vi "HMI Panel.vi"() -> ()   [LabVIEW 2014]
uses:
  <vilib>/Platform/TimedLoop/XDataNode/timing_clust.ctl
  <vilib>/Platform/TimedLoop/XDataNode/nitl_modes.ctl
  <vilib>/Platform/TimedLoop/XDataNode/wakeup.ctl
  <vilib>/Utility/inputDevices.llb/closeJoystick.vi
  <vilib>/Utility/inputDevices.llb/joystickAcquire.vi
  <vilib>/Platform/TimedLoop/XDataNode/XDataNode.xnode
  <vilib>/Platform/TimedLoop/XDataNode/XDNodeRunTimeDep.lvlib
panel:
  out "error out 2":errorcluster
  out "data out 2":string
  out "data out":string
  out "Period":i64
  out "Finished Late? [i-1]":bool
  out "String":string
  out "error out 3":errorcluster
  out "error out":errorcluster
  in  "error in":errorcluster
  in  "error in":errorcluster
  in  "Activate Joystick":bool=TRUE
  in  "Activate Oculus Rift":bool
  in  "?":enum32{"Logiteck Joystick", "Oculus Rift"}(tab)
  in  "?":dbl
  in  "?":dbl
  in  "?":dbl
  out "Vertical":dbl(slide) scale=-100.0..100.0
  out "?":cluster{dbl[], dbl[]}[](graph)
  out "Yaw":dbl(slide) scale=-100.0..100.0
  out "?":dbl(knob) scale=0.0..360.0
  out "Joystick Status":bool
  in  "Joystick Selector":u16(ring)=1 items=["Logitech Freedom 2.4 USB"]
  out "z":dbl(slide) scale=-1.5..1.5
  out "y":dbl(slide) scale=-1.5..1.5
  out "x":dbl(slide) scale=-1.5..1.5
  in  "Operation Mode":u16(ring)=1 items=["Disabled", "Standard"]
  in  "Port Joyst.TCP":u16=6340
  out "Oculus Rift Status":bool
  in  "SYA":dbl(slide)=1.0 scale=0.0..1.0
  in  "SZR":dbl(slide)=1.0 scale=0.0..1.0
  in  "SZA":dbl(slide)=1.0 scale=0.0..1.0
  in  "SXA":dbl(slide)=1.0 scale=0.0..1.0
  out "Error Out":errorcluster
  in  "DZZR":i32(slide)=20 scale=0.0..100.0
  in  "DZZA":i32(slide)=20 scale=0.0..100.0
  in  "DZYA":i32(slide)=10 scale=0.0..100.0
  in  "DZXA":i32(slide)=10 scale=0.0..100.0
  in  "InvZA":bool=TRUE
  in  "InvYA":bool
  in  "InvXA":bool
  in  "stop":bool
  in  "Joystick Button Ref":refnum<vi>
  in  "TCPConRef":refnum<k5>
  out "direction info":T1
  out "button info":T2
  out "axis info":T3
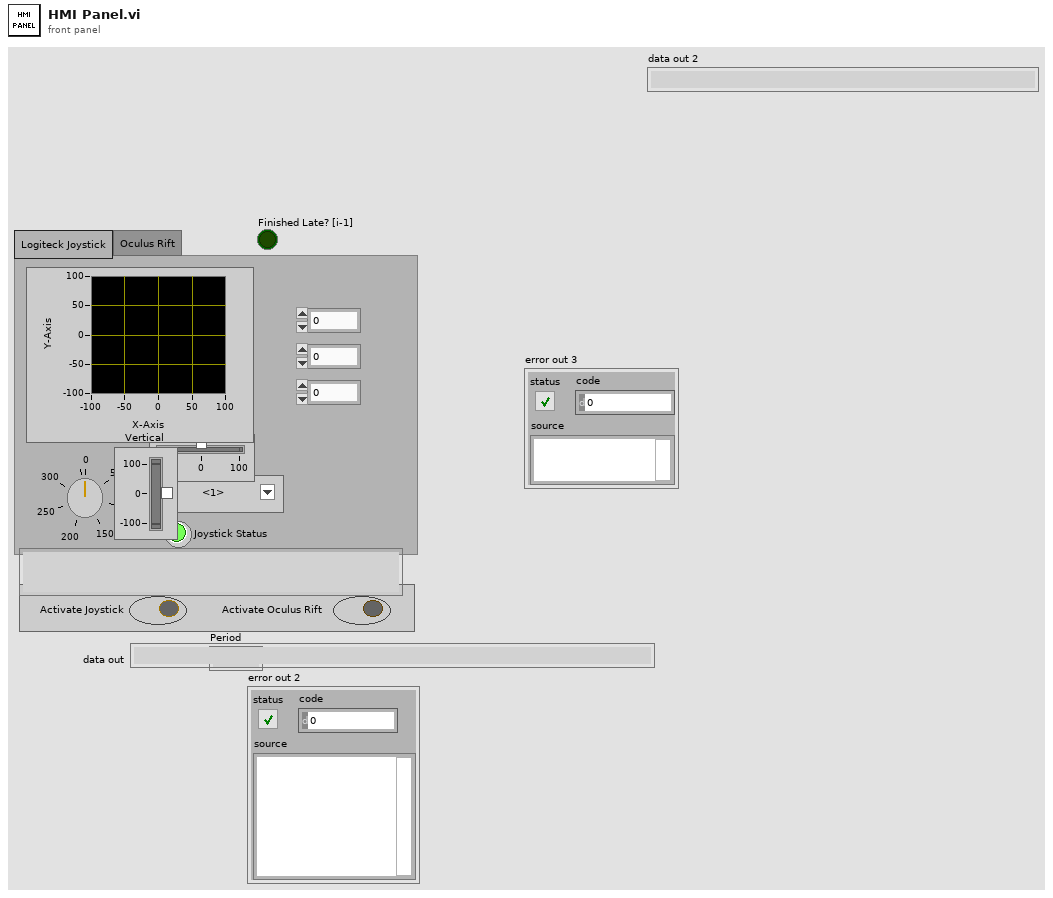
[diagram p1: front panel]
types:
  T1 = cluster{"pov 1":i32, "pov 2":i32, "pov 3":i32, "pov 4":i32}
  T2 = cluster{"button 1":bool, "button 2":bool, "button 3":bool, "button 4":bool, "button 5":bool, "button 6":bool, "button 7":bool, "button 8":bool, "button 9":bool, "button 10":bool, "button 11":bool, "button 12":bool, "button 13":bool, "button 14":bool, "button 15":bool, "button 16":bool, "button 17":bool, "button 18":bool, "button 19":bool, "button 20":bool, "button 21":bool, "button 22":bool, "button 23":bool, "button 24":bool, "button 25":bool, "button 26":bool, "button 27":bool, "button 28":bool, "button 29":bool, "button 30":bool, "button 31":bool, "button 32":bool}
  T3 = cluster{"X axis":i32, "Y axis":i32, "Z axis":i32, "X axis rotation":i32, "Y axis rotation":i32, "Z axis rotation":i32, "U axis":i32, "V axis":i32}
  T4 = typedef "XDNodeRunTimeDep.lvlib/timing_clust.ctl" = cluster{"Expected End [f-1]":u64, "Actual End [f-1]":u64, "Finished Late? [f-1]":bool, "Expected End [i-1]":u64, "Actual End [i-1]":u64, "Finished Late? [i-1]":bool, "Expected Start [i]":u64, "Actual Start [i]":u64, "Expected Start [f]":u64, "Actual Start [f]":u64, "Source Name":string, "Structure Name":string, "Period":i64, "Deadline":i64, "Offset":i64, "Start":i64, "Priority":i32, "Timeout":i32, "Mode":T5, "Wakeup Reason":T6, "Error":errorcluster, "Source Type":string, "Secondary Source Type":string, "Global End Time":u64, "Global Start Time":u64, "Frame Duration":u64, "Iteration Duration":u64, "Assigned CPU":i32, "I/O Scan Engine Mode":u32}
  T5 = typedef "XDNodeRunTimeDep.lvlib/nitl_modes.ctl" = enum32{"No Change", "Process missed periods, maintain original phase", "Discard missed periods, maintain original phase", "Process missed periods, ignore original phase", "Discard missed periods, ignore original phase"}
  T6 = typedef "XDNodeRunTimeDep.lvlib/wakeup.ctl" = enum32{"Normal", "Aborted", "Asynchronous wakeup", "Timing source error", "Timed loop error", "Timeout"}
  T7 = cluster{"axes total":u32, "buttons total":u32, "pov total":u32, "device name":string}[]
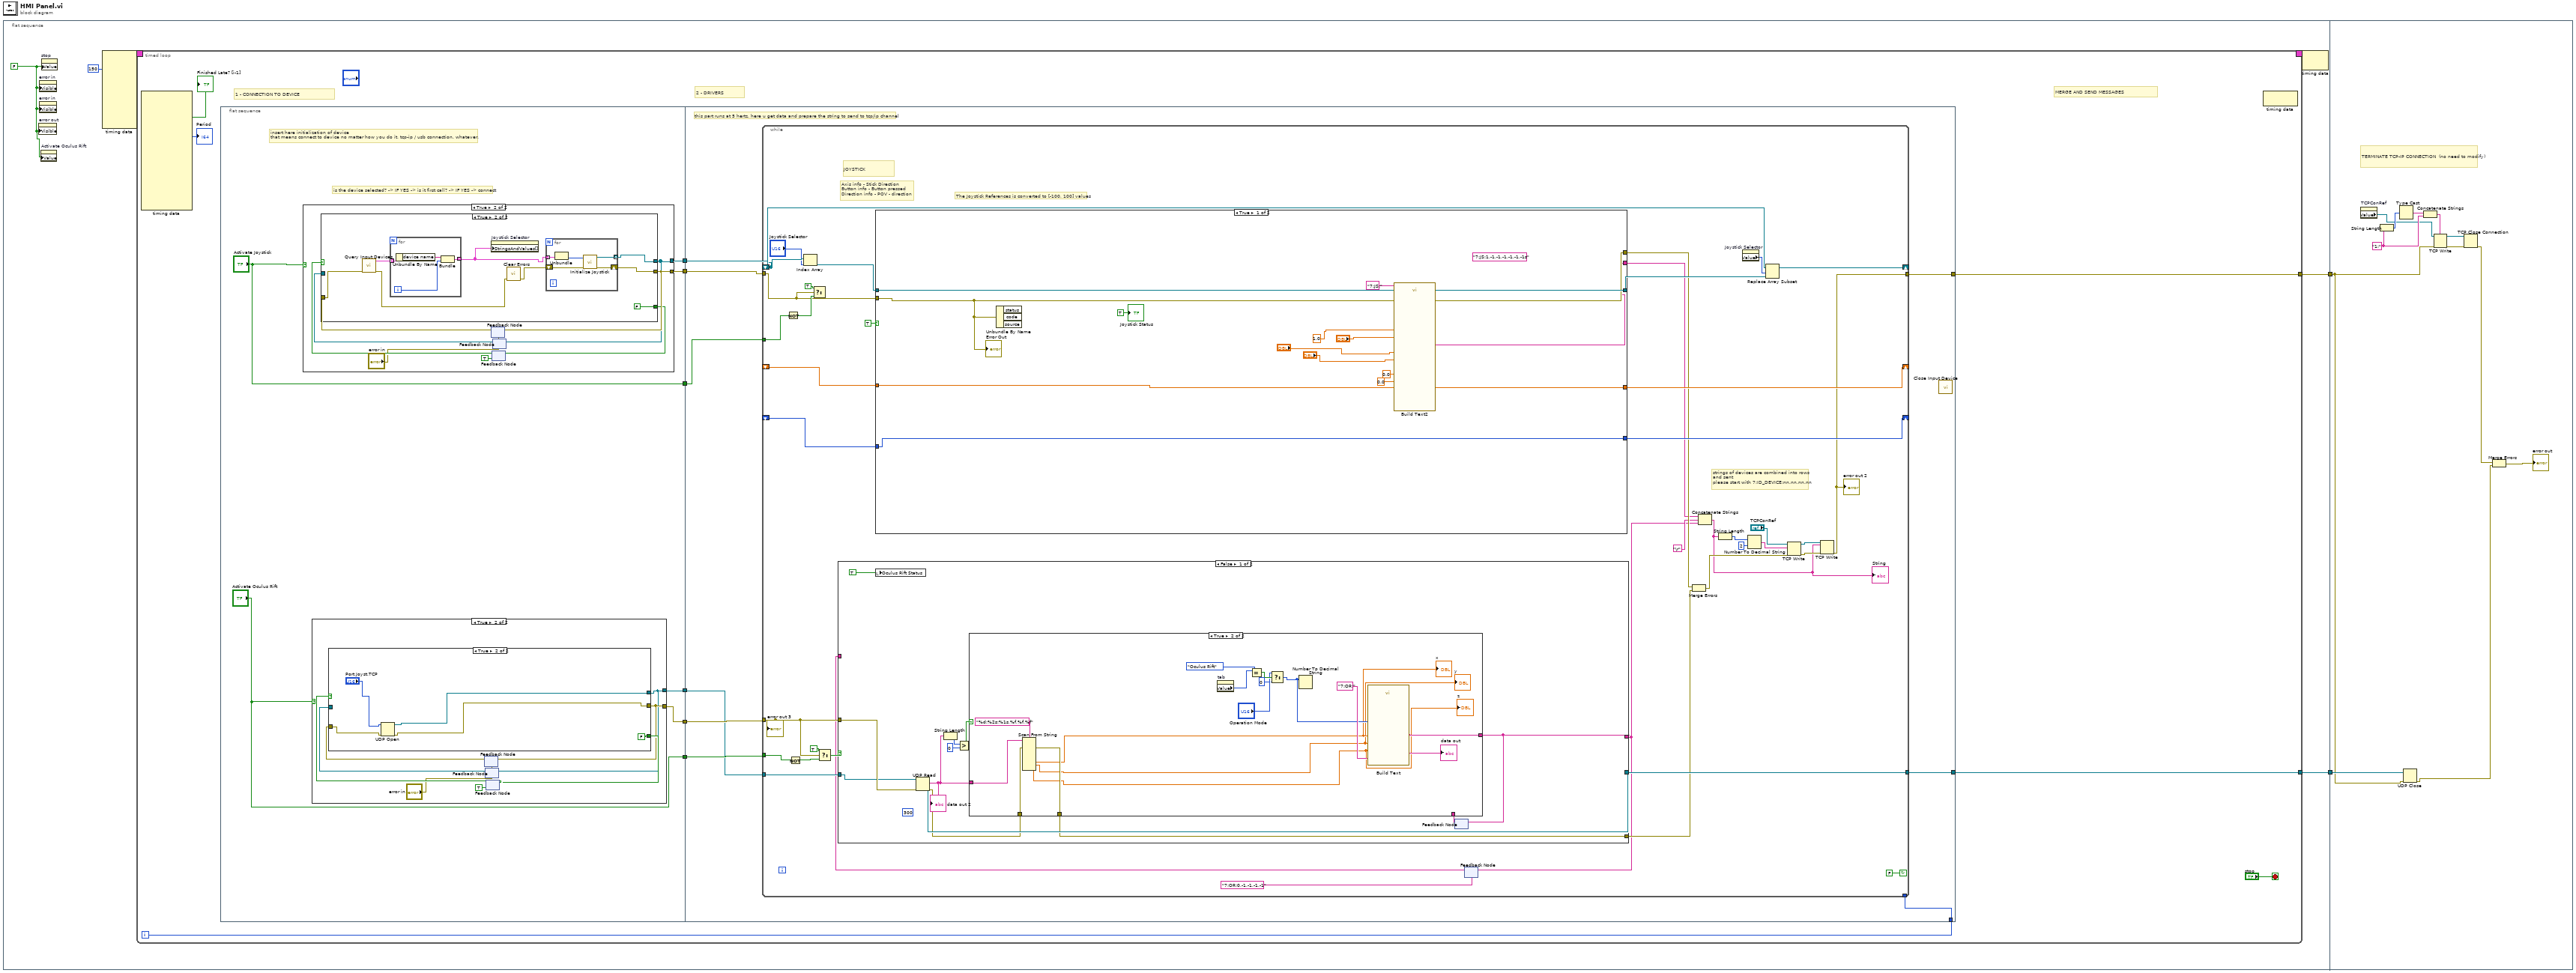
[diagram p0: block diagram]
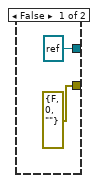
[diagram p2: hidden frame]
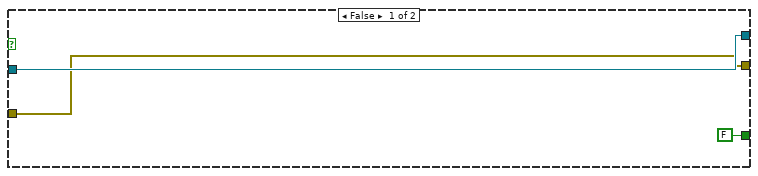
[diagram p3: hidden frame]
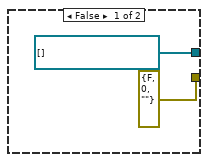
[diagram p4: hidden frame]
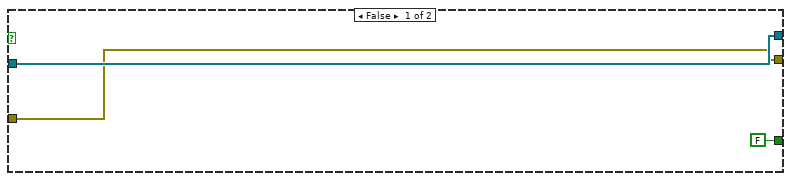
[diagram p5: hidden frame]
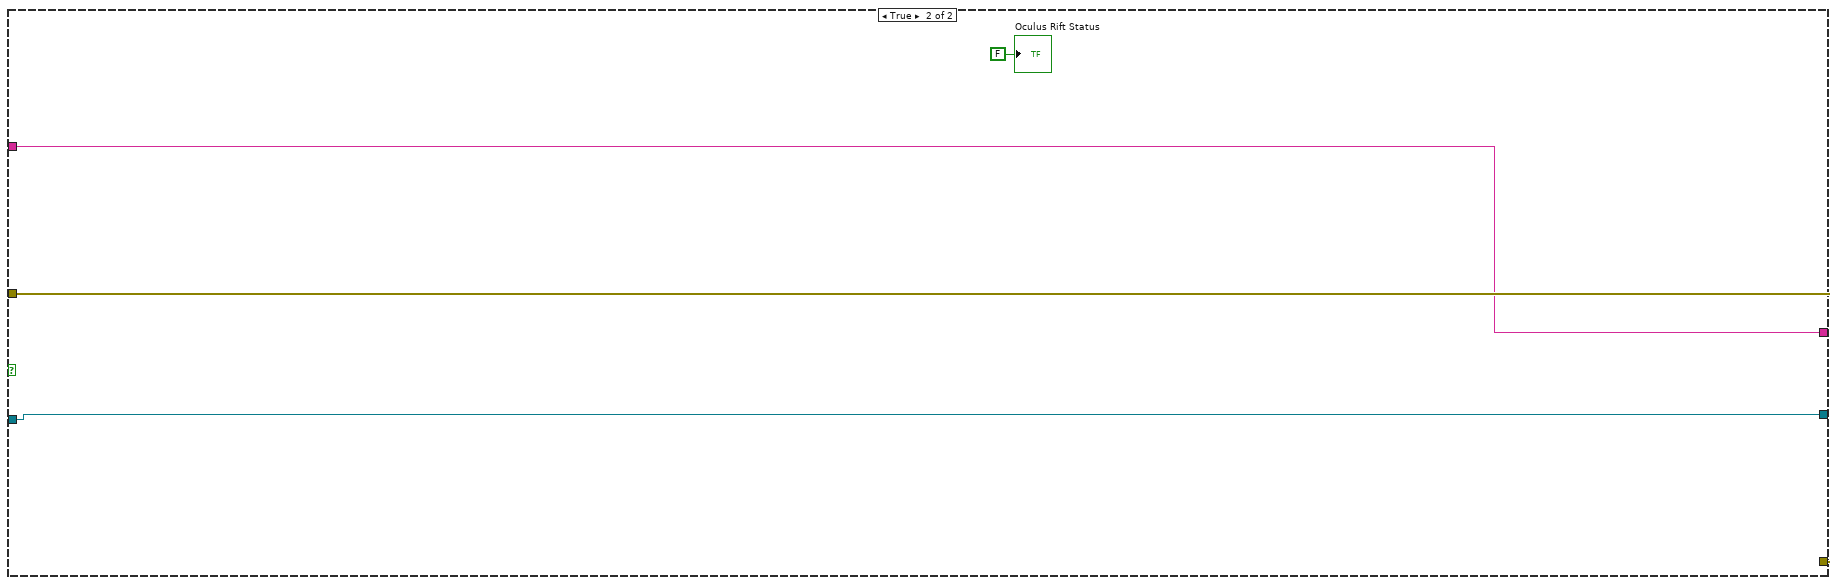
[diagram p7: hidden frame]
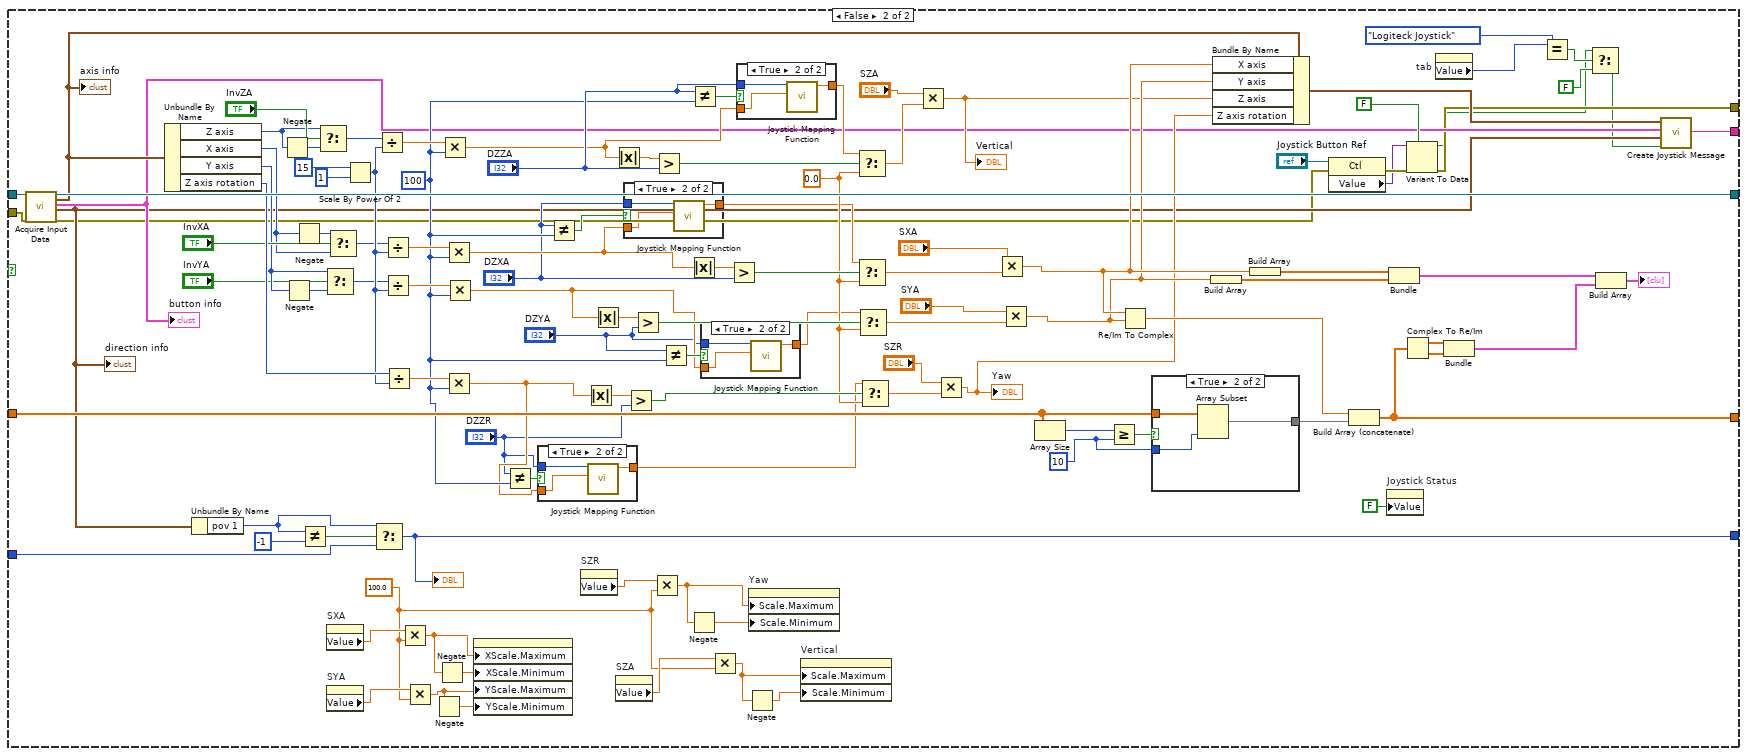
[diagram p8: hidden frame]
diagram:
  n1 = flat-sequence {
    tunnel: [w5] -> w2
    tunnel: [w4] -> w1
    tunnel: w2 -> [w310]
    tunnel: w1 -> [w309]
    frame #0 {
      w3 = FALSE
      n2 = property on="error out" class="Clust (strict)"("Visible"=w3) -> ()  [unwired: 2 in, 2 out]
      n3 = property on="error in" class="Clust (strict)"("Visible"=w3) -> ()  [unwired: 2 in, 2 out]
      n4 = property on="error in" class="Clust (strict)"("Visible"=w3) -> ()  [unwired: 2 in, 2 out]
      n5 = property on="Activate Oculus Rift" class="Bool (strict)"("Value"=w3) -> ()  [unwired: 2 in, 2 out]
      n6 = property on="stop" class="Bool (strict)"("Value"=w3) -> ()  [unwired: 2 in, 2 out]
      n7 = node-c288(i64 150 ("Period")) -> (w8:T4)  [unwired: 9 in]
      n8 = timed-loop {
        timing: w8 -> [_]
        timing-out: [_] -> w7
        tunnel: [w14] -> w5
        tunnel: [w13] -> w4
        i -> [w12]
        stop <- "stop" stop-if-true
        # "MERGE AND SEND MESSAGES"
        # "2 - DRIVERS"
        # "1 - CONNECTION TO DEVICE"
        n9 = node-c288() -> (→"Finished Late? [i-1]":bool, →"Period":i64)  [unwired: 1 in, 15 out]
        n10 = flat-sequence {
          tunnel: [w26] -> w20
          tunnel: [w25] -> w19
          tunnel: ["Activate Joystick"] -> w17
          tunnel: [w23] -> w16
          tunnel: ["Activate Oculus Rift"] -> w15
          tunnel: [w21] -> w9
          tunnel: w20 -> [w83]
          tunnel: w19 -> [w77]
          tunnel: w17 -> [w82]
          tunnel: w16 -> [w81]
          tunnel: w15 -> [w80]
          tunnel: [w79] -> w14
          tunnel: [w78] -> w13
          tunnel: w12 -> [w76]
          tunnel: w9 -> [w75]
          frame #0 {
            # "insert here initialization of device \nthat means connect to device no matter how you do it. tcp-ip / usb connection. whatever."
            # "is the device selected? -> IF YES -> is it first call? -> IF YES -> connect"
            n11 = case shown="True" "Activate Joystick" {
              tunnel: [w46 w52] -> w26
              tunnel: [errorcluster {"status"=FALSE, "code"=0, "source"=""} ("error out") w53] -> w25
              frame False {
                w46 = refnum<k1>[] [] items=["JOYSTICK"]
              }
              frame True {
                n12 = feedback #1("error in") -> (w51:errorcluster)
                n13 = feedback #2(TRUE) -> (w49:bool)
                n14 = feedback #3() -> (w54:refnum<k1>[])  [unwired: 1 in]
                n15 = case shown="True" w49 {
                  tunnel: [w57 w64] -> w52
                  tunnel: [w56 w63] -> w53
                  tunnel: w54 -> [w57 _]
                  tunnel: w51 -> [w56 w58]
                  tunnel: [FALSE FALSE] -> w50
                  frame False {
                  }
                  frame True {
                    n16 = call <vilib>:"Query Input Devices.vi"("error in (no error)"=w58) -> ("error out"=w61:errorcluster, "joystick info"=w60:T7)  [unwired: 7 in, 2 out]
                    n17 = for {
                      tunnel: w60 -> [w74] mode=indexing
                      tunnel: [w71] -> w65 mode=indexing
                      i -> [w72]
                      n18 = Unbundle By Name(w74) -> ("device name"=w73:string)
                      n19 = Bundle("device name"=w73, w72) -> (w71:cluster{"device name":string, i32})  [unwired: 1 in]
                    }
                    n20 = property on="Joystick Selector" class="Ring (strict)"("StringsAndValues[]"=w65) -> ()  [unwired: 2 in, 2 out]
                    n21 = call <vilib>:"Clear Errors.vi"("error in (no error)"=w61) -> ("error out"=w59:errorcluster)  [unwired: 5 in, 1 out]
                    n22 = for {
                      tunnel: w65 -> [w67] mode=indexing
                      tunnel: [w70] -> w64 mode=indexing
                      shift-right: [w68] -> w63
                      shift-left: w59 -> [w69]
                      n23 = Unbundle(w67) -> (w66:i32)  [unwired: 1 out]
                      n24 = call <vilib>:"Initialize Joystick.vi"("error in (no error)"=w69, "device index"=w66) -> ("error out"=w68:errorcluster, "device ID"=w70:refnum<k1>)  [unwired: 8 in]
                    }
                  }
                }
                n25 = feedback-in #1(w53) -> ()
                n26 = feedback-in #2(w50) -> ()
                n27 = feedback-in #3(w52) -> ()
              }
            }
            n28 = case shown="True" "Activate Oculus Rift" {
              tunnel: [errorcluster {"status"=FALSE, "code"=0, "source"=""} ("error out") w31] -> w23
              tunnel: [refnum<k16> refnum ("port") w29] -> w21
              frame False {
              }
              frame True {
                n29 = feedback #4("error in") -> (w32:errorcluster)
                n30 = feedback #5() -> (w33:refnum<k16>)  [unwired: 1 in]
                n31 = feedback #6(TRUE) -> (w35:bool)
                n32 = case shown="True" w35 {
                  tunnel: [w39 w41] -> w29
                  tunnel: [w38 w42] -> w31
                  tunnel: w33 -> [w39 _]
                  tunnel: w32 -> [w38 w43]
                  tunnel: [FALSE FALSE] -> w34
                  frame False {
                  }
                  frame True {
                    n33 = UDP Open(8:w43, 11:"Port Joyst.TCP") -> (port=w41:refnum<k16>, 0:w42:errorcluster)  [unwired: 3 in, 1 out]
                  }
                }
                n34 = feedback-in #4(w31) -> ()
                n35 = feedback-in #5(w29) -> ()
                n36 = feedback-in #6(w34) -> ()
              }
            }
          }
          frame #1 {
            # "this part runs at 5 hertz. here u get data and prepare the string to send to tcp/ip channel"
            n37 = while {
              shift-right: [w117] -> _
              shift-left: w83 -> [w118]
              shift-right: [w122] -> _
              shift-left: _ -> [w121]
              shift-right: [w119] -> _
              shift-left: _ -> [w120]
              tunnel: w82 -> [w113]
              tunnel: w81 -> [w106]
              tunnel: w80 -> [w107]
              tunnel: [w105] -> w79
              tunnel: [w104] -> w78
              tunnel: w77 -> [w103]
              tunnel: w76 -> [_]
              tunnel: w75 -> [w100]
              stop <- FALSE continue-if-true
              # "strings of devices are combined into rows\nand sent\nplease start with 7:ID_DEVICE:nn,nn,nn,nn"
              # "JOYSTICK"
              # "The Joystick References is converted to [-100, 100] values"
              # "Axis info - Stick Direction\nButton info - Button pressed\nDirection info - POV - direction"
              n38 = Not(x=w113) -> (.not. x?=w112:bool)
              n39 = Not(x=w107) -> (.not. x?=w108:bool)
              n40 = Index Array(array=w118, index="Joystick Selector") -> (element=w110:refnum<k1>)
              n41 = Select(t=TRUE, s=w103, f=w112) -> ()  [unwired: 1 out]
              n42 = Select(t=TRUE, s=w106, f=w108) -> (s? t:f=w89:bool)
              n43 = case shown="True" TRUE {
                tunnel: w110 -> [w168 w279]
                tunnel: [w168 w278] -> w115
                tunnel: [w166 w264] -> w122
                tunnel: w121 -> [w166 w263]
                tunnel: w120 -> [w167 w259]
                tunnel: [w167 w254] -> w119
                tunnel: [w164 w178] -> w102
                tunnel: [w156 w177] -> w92
                tunnel: w103 -> [w164 w169]
                frame True {
                  (unwired) "7:JS:1,-1,-1,-1,-1,-1,-1s" ("Message Output")
                  n44 = Unbundle By Name(w164) -> ()  [unwired: 3 out]
                  n45 = call "Build Text2"("Beginning Text"="7:JS:", "Button Command"=0.0, "Joystick Status"=1.0, "X-Axis"="?", "Y-Axis"="?", "Z-Rotation"="?", "POV"=0.0) -> ("Result"=w156:string)  [unwired: 7 in, 1 out]
                  "Joystick Status" <- TRUE ("Joystick Status")
                  "Error Out" <- w164
                }
                frame False {
                  w184 = 100.0
                  w228 = 0.0
                  w258 = 10
                  w216 = 100
                  n46 = call-poly <vilib>:"Acquire Input Data.vi"("device ID"=w279, "error in (no error)"=w169) -> ("device ID"=w278:refnum<k1>, "axis info"=w237:T3, "button info"=w180:T2, "direction info"=w179:T1, "error out"=w176:errorcluster)  [unwired: 13 in]
                  "axis info" <- w237
                  "button info" <- w180
                  "direction info" <- w179
                  n47 = Unbundle By Name(w237) -> ("Z axis"=w248:i32, "X axis"=w243:i32, "Y axis"=w240:i32, "Z axis rotation"=w270:i32)
                  n48 = Unbundle By Name(w179) -> ("pov 1"=w265:i32)
                  n49 = Negate(x=w248) -> (-x=w249:i32)
                  n50 = Negate(x=w240) -> (-x=w242:i32)
                  n51 = Negate(x=w243) -> (-x=w244:i32)
                  n52 = Not Equal?(x=w265, y=-1) -> (x != y?=w266:bool)
                  n53 = Select(t=w248, s="InvZA", f=w249) -> (s? t:f=w247:i32)
                  n54 = Select(t=w240, s="InvYA", f=w242) -> (s? t:f=w241:i32)
                  n55 = property on="SXA" class="Slide (strict)"() -> ("Value"=w194:dbl)  [unwired: 2 in, 2 out]
                  n56 = property on="SYA" class="Slide (strict)"() -> ("Value"=w193:dbl)  [unwired: 2 in, 2 out]
                  n57 = Select(t=w244, s="InvXA", f=w243) -> (s? t:f=w246:i32)
                  n58 = Scale By Power Of 2(n=15, x=1) -> (x*2^n=w269:i32)
                  n59 = Select(t=w265, s=w266, f=w263) -> (s? t:f=w264:i32)
                  "?" <- w264
                  n60 = Divide(x=w247, y=w269) -> (x/y=w275:dbl)
                  n61 = Divide(x=w246, y=w269) -> (x/y=w274:dbl)
                  n62 = Divide(x=w241, y=w269) -> (x/y=w273:dbl)
                  n63 = Divide(x=w270, y=w269) -> (x/y=w268:dbl)
                  n64 = Multiply(x=w194, y=w184) -> (x*y=w189:dbl)
                  n65 = Multiply(x=w193, y=w184) -> (x*y=w191:dbl)
                  n66 = Negate(x=w191) -> (-x=w192:dbl)
                  n67 = Negate(x=w189) -> (-x=w190:dbl)
                  n68 = Multiply(x=w275, y=w216) -> (x*y=w221:dbl)
                  n69 = Multiply(x=w274, y=w216) -> (x*y=w215:dbl)
                  n70 = Multiply(x=w268, y=w216) -> (x*y=w209:dbl)
                  n71 = Multiply(x=w273, y=w216) -> (x*y=w212:dbl)
                  n72 = property class="XYGraph (strict)"("XScale.Maximum"=w189, "XScale.Minimum"=w190, "YScale.Maximum"=w191, "YScale.Minimum"=w192) -> ()  [unwired: 2 in, 2 out]
                  n73 = Not Equal?(x="DZZR", y=w216) -> (x != y?=w219:bool)
                  n74 = case shown="True" w219 {
                    tunnel: "DZZR" -> [_ w282]
                    tunnel: w209 -> [w280 w283]
                    tunnel: [w280 w281] -> w207
                    frame False {
                    }
                    frame True {
                      n75 = call "Joystick Mapping Function.vi"("Gain"=w283, "Dead Zone"=w282) -> ("Gain Out"=w281:dbl)  [unwired: 9 in]
                    }
                  }
                  n76 = Not Equal?(x="DZXA", y=w216) -> (x != y?=w217:bool)
                  n77 = property on="SZR" class="Slide (strict)"() -> ("Value"=w188:dbl)  [unwired: 2 in, 2 out]
                  n78 = Absolute Value(x=w209) -> (abs(x)=w232:dbl)
                  n79 = Absolute Value(x=w212) -> (abs(x)=w234:dbl)
                  n80 = Absolute Value(x=w221) -> (abs(x)=w236:dbl)
                  n81 = property on="SZA" class="Slide (strict)"() -> ("Value"=w185:dbl)  [unwired: 2 in, 2 out]
                  n82 = case shown="True" w217 {
                    tunnel: "DZXA" -> [_ w290]
                    tunnel: w215 -> [w288 w291]
                    tunnel: [w288 w289] -> w213
                    frame False {
                    }
                    frame True {
                      n83 = call "Joystick Mapping Function.vi"("Gain"=w291, "Dead Zone"=w290) -> ("Gain Out"=w289:dbl)  [unwired: 9 in]
                    }
                  }
                  n84 = Greater?(x=w232, y="DZZR") -> (0:w231:bool)
                  n85 = Greater?(x=w234, y="DZYA") -> (0:w233:bool)
                  n86 = Multiply(x=w188, y=w184) -> (x*y=w187:dbl)
                  n87 = Greater?(x=w236, y="DZZA") -> (0:w235:bool)
                  n88 = Not Equal?(x="DZYA", y=w216) -> (x != y?=w218:bool)
                  n89 = Absolute Value(x=w215) -> (abs(x)=w230:dbl)
                  n90 = Negate(x=w187) -> (-x=w186:dbl)
                  n91 = Not Equal?(x="DZZA", y=w216) -> (x != y?=w223:bool)
                  n92 = case shown="True" w218 {
                    tunnel: "DZYA" -> [_ w286]
                    tunnel: w212 -> [w284 w287]
                    tunnel: [w284 w285] -> w211
                    frame False {
                    }
                    frame True {
                      n93 = call "Joystick Mapping Function.vi"("Gain"=w287, "Dead Zone"=w286) -> ("Gain Out"=w285:dbl)  [unwired: 9 in]
                    }
                  }
                  n94 = Multiply(x=w185, y=w184) -> (x*y=w183:dbl)
                  n95 = Greater?(x=w230, y="DZXA") -> (0:w229:bool)
                  n96 = case shown="True" w223 {
                    tunnel: "DZZA" -> [_ w294]
                    tunnel: w221 -> [w292 w295]
                    tunnel: [w292 w293] -> w220
                    frame False {
                    }
                    frame True {
                      n97 = call "Joystick Mapping Function.vi"("Gain"=w295, "Dead Zone"=w294) -> ("Gain Out"=w293:dbl)  [unwired: 9 in]
                    }
                  }
                  n98 = Negate(x=w183) -> (-x=w182:dbl)
                  n99 = property on="Yaw" class="Slide (strict)"("Scale.Maximum"=w187, "Scale.Minimum"=w186) -> ()  [unwired: 2 in, 2 out]
                  n100 = property on="Vertical" class="Slide (strict)"("Scale.Maximum"=w183, "Scale.Minimum"=w182) -> ()  [unwired: 2 in, 2 out]
                  n101 = Select(t=w220, s=w235, f=w228) -> (s? t:f=w196:dbl)
                  n102 = Select(t=w213, s=w229, f=w228) -> (s? t:f=w205:dbl)
                  n103 = Select(t=w211, s=w233, f=w228) -> (s? t:f=w202:dbl)
                  n104 = Select(t=w207, s=w231, f=w228) -> (s? t:f=w199:dbl)
                  n105 = Multiply(x="SZA", y=w196) -> (x*y=w195:dbl)
                  "Vertical" <- w195
                  n106 = Multiply(x="SZR", y=w199) -> (x*y=w198:dbl)
                  "Yaw" <- w198
                  n107 = Multiply(x="SXA", y=w205) -> (x*y=w204:dbl)
                  n108 = Multiply(x="SYA", y=w202) -> (x*y=w201:dbl)
                  n109 = Array Size(array=w259) -> (size(s)=w261:i32)
                  n110 = Greater Or Equal?(x=w261, y=w258) -> (x >= y?=w260:bool)
                  n111 = Re/Im To Complex(1:w201, 2:w204) -> (0:w262:cdb)
                  n112 = case shown="True" w260 {
                    tunnel: w259 -> [w296 w299]
                    tunnel: w258 -> [_ w298]
                    tunnel: [w296 w297] -> w257
                    frame False {
                    }
                    frame True {
                      n113 = Array Subset(array=w299, length=w298) -> (w297:cdb[])  [unwired: 1 in]
                    }
                  }
                  n114 = Build Array(w201) -> (w252:dbl[])
                  n115 = Bundle By Name(cluster=w237, "X axis"=w204, "Y axis"=w201, "Z axis"=w195, "Z axis rotation"=w198) -> (w181:T3)
                  n116 = Build Array(w204) -> (w253:dbl[])
                  n117 = property class="Ctl"(reference="Joystick Button Ref", error in=w176) -> (error out=w226:errorcluster, "Value"=w225:variant)  [unwired: 1 out]
                  n118 = Build Array (concatenate)(w262, w257) -> (w254:cdb[])
                  n119 = property on="Joystick Status" class="Bool (strict)"("Value"=FALSE ("Joystick Status")) -> ()  [unwired: 2 in, 2 out]
                  n120 = Bundle(w253, w252) -> (w272:cluster{dbl[], dbl[]})  [unwired: 1 in]
                  n121 = Complex To Re/Im(x + iy=w254) -> (x=w256:dbl[], y=w255:dbl[])
                  n122 = Variant To Data(error in=w226, type=FALSE, Variant=w225) -> (data=w171:bool, error out=w178:errorcluster)
                  n123 = property on="tab" class="TabCtl (strict)"() -> ("Value"=w173:enum32{"Logiteck Joystick", "Oculus Rift"})  [unwired: 2 in, 2 out]
                  n124 = Bundle(w256, w255) -> (w251:cluster{dbl[], dbl[]})  [unwired: 1 in]
                  n125 = Equal?(x=w173, y=enum32{"Logiteck Joystick", "Oculus Rift"}."Logiteck Joystick") -> (x = y?=w174:bool)
                  n126 = Select(t=w171, s=w174, f=FALSE ("x = y?")) -> (s? t:f=w170:bool)
                  n127 = Build Array(w272, w251) -> (→"?":cluster{dbl[], dbl[]}[])
                  n128 = call "Create Joystick Message.vi"("Joystick Active"=w170, "direction info"=w179, "button info"=w180, "axis info"=w181) -> ("Message Output"=w177:string)  [unwired: 7 in]
                }
              }
              n129 = feedback #7("7:OR:0,-1,-1,-1,-1") -> (w86:string)
              n130 = case shown="False" w89 {
                tunnel: [w124 w152] -> w85
                tunnel: w106 -> [w133 w155]
                tunnel: [w129 w155] -> w101
                tunnel: [w131 w153] -> w105
                tunnel: w100 -> [w132 w153]
                tunnel: w86 -> [_ w152]
                frame False {
                  (unwired) 300
                  n131 = local write "Oculus Rift Status"(TRUE ("Joystick Status")) -> ()
                  n132 = UDP Read(connection ID=w132, 8:w133) -> (data out=w128:string, error out=w130:errorcluster, 3:w131:refnum<k16>)  [unwired: 2 in, 2 out]
                  "data out 2" <- w128
                  n133 = String Length(string=w128) -> (length=w127:i32)
                  n134 = Greater?(x=w127, y=0) -> (0:w125:bool)
                  n135 = feedback #8() -> (w123:string)  [unwired: 1 in]
                  n136 = case shown="True" w125 {
                    tunnel: w128 -> [_ w145]
                    tunnel: [w136 w142] -> w124
                    tunnel: w130 -> [w135 w141]
                    tunnel: [w135 w140] -> w129
                    tunnel: w123 -> [w136 _]
                    frame False {
                    }
                    frame True {
                      n137 = Scan From String(format string="%d:%2s:%1s,%f,%f,%f", input string=w145, error in=w141) -> (error out=w140:errorcluster, output 4=w139:dbl, output 5=w138:dbl, output 6=w137:dbl)  [unwired: 10 in, 2 out]
                      "x" <- w139
                      "y" <- w138
                      "z" <- w137
                      n138 = property on="tab" class="TabCtl (strict)"() -> ("Value"=w151:enum32{"Logiteck Joystick", "Oculus Rift"})  [unwired: 2 in, 2 out]
                      n139 = Equal?(x=w151, y=enum32{"Logiteck Joystick", "Oculus Rift"}."Oculus Rift") -> (x = y?=w149:bool)
                      n140 = Select(t="Operation Mode", s=w149, f=u16 0) -> (s? t:f=w143:u16)
                      n141 = Number To Decimal String(number=w143) -> ()  [unwired: 1 in, 1 out]
                      n142 = call "Build Text"("Beginning Text"="7:OR:", "val3"=w137, "ORStatus"=w143, "val1"=w139, "val2"=w138) -> ("Result"=w142:string)  [unwired: 9 in, 1 out]
                      "data out" <- w142
                    }
                  }
                  n143 = feedback-in #8(w124) -> ()
                }
                frame True {
                  "Oculus Rift Status" <- FALSE ("Joystick Status")
                }
              }
              n144 = feedback-in #7(w85) -> ()
              n145 = Merge Errors(w102, w101) -> (w95:errorcluster)
              n146 = Concatenate Strings(w92, "\r", w85) -> (w87:string)
              "String" <- w87
              n147 = String Length(string=w87) -> (length=w99:i32)
              n148 = property on="Joystick Selector" class="Ring (strict)"() -> ("Value"=w116:u16)  [unwired: 2 in, 2 out]
              n149 = Number To Decimal String(number=w99, width (-)=i16 2) -> (decimal integer string=w98:string)
              n150 = Replace Array Subset(array=w118, new element=w115, index=w116) -> (w117:refnum<k1>[])
              n151 = TCP Write(connection ID="TCPConRef", data in=w98, error in (no error)=w95) -> (connection ID out=w96:refnum<k5>, error out=w94:errorcluster)  [unwired: 1 in, 1 out]
              n152 = TCP Write(connection ID=w96, data in=w87, error in (no error)=w94) -> (error out=w104:errorcluster)  [unwired: 1 in, 2 out]
              "error out 2" <- w104
              "error out 3" <- w106
            }
            n153 = call-poly <vilib>:"Close Input Device.vi"() -> ()  [unwired: 10 in, 1 out]
          }
        }
        n154 = node-c288() -> ()  [unwired: 1 in, 1 out]
      }
      n155 = node-c288(w7) -> ()  [unwired: 1 out]
    }
    frame #1 {
      w317 = "1:"
      # "TERMINATE TCP-IP CONNECTION  (no need to modify)"
      n156 = property on="TCPConRef" class="Ref (strict)"() -> ("Value"=w315:refnum<k5>)  [unwired: 2 in, 2 out]
      n157 = String Length(string=w317) -> (length=w319:i32)
      n158 = Type Cast(x=w319) -> (*(type *) &x=w318:string)  [unwired: 1 in]
      n159 = UDP Close(connection ID=w310, 8:w309) -> (error out=w308:errorcluster)  [unwired: 1 out]
      n160 = Concatenate Strings(w318, w317) -> (w316:string)
      n161 = TCP Write(connection ID=w315, data in=w316, error in (no error)=w309) -> (connection ID out=w314:refnum<k5>, error out=w313:errorcluster)  [unwired: 1 in, 1 out]
      n162 = TCP Close Connection(connection ID=w314, error in (no error)=w313) -> (error out=w312:errorcluster)  [unwired: 1 in, 1 out]
      n163 = Merge Errors(w312, w308) -> (→"error out":errorcluster)
    }
  }
